vi "Build DashBoard Data.vi"(8 "finish":bool, 11 "Dashboard Enables":T3={"Analog Module 1"=[TRUE, TRUE, TRUE, TRUE, TRUE, TRUE, TRUE, TRUE], "Analog Module 2"=[FALSE, FALSE, FALSE, FALSE, FALSE, FALSE, FALSE, FALSE], "Digital Module 1"=TRUE, "Digital Module 2"=FALSE, "Solenoid Module"=TRUE}) -> ()   [LabVIEW 2011]
doc: "This VI builds data and sends it back to the dashboard PC program. By default it sends back the raw values for the first analog, digital, and solenoid module. Modify it to send back the data you want to view. Consider adding higher level data to the Dashboard Datatype.ctl and to this VI. Then update the Dashboard to display the data however you like.\n\nThis software is licensed. Open the labview\\readme\\WPI Robotics Library Open Source License.txt file for more information."
uses:
  DashboardEnable.ctl
  Dashboard Datatype.ctl
  <vilib>/Rock Robotics/WPI/DriverStation/WPI_DriverStationDigitalData.ctl
  Robot Global Data.vi
panel:
  out "Dashboard Data":T1
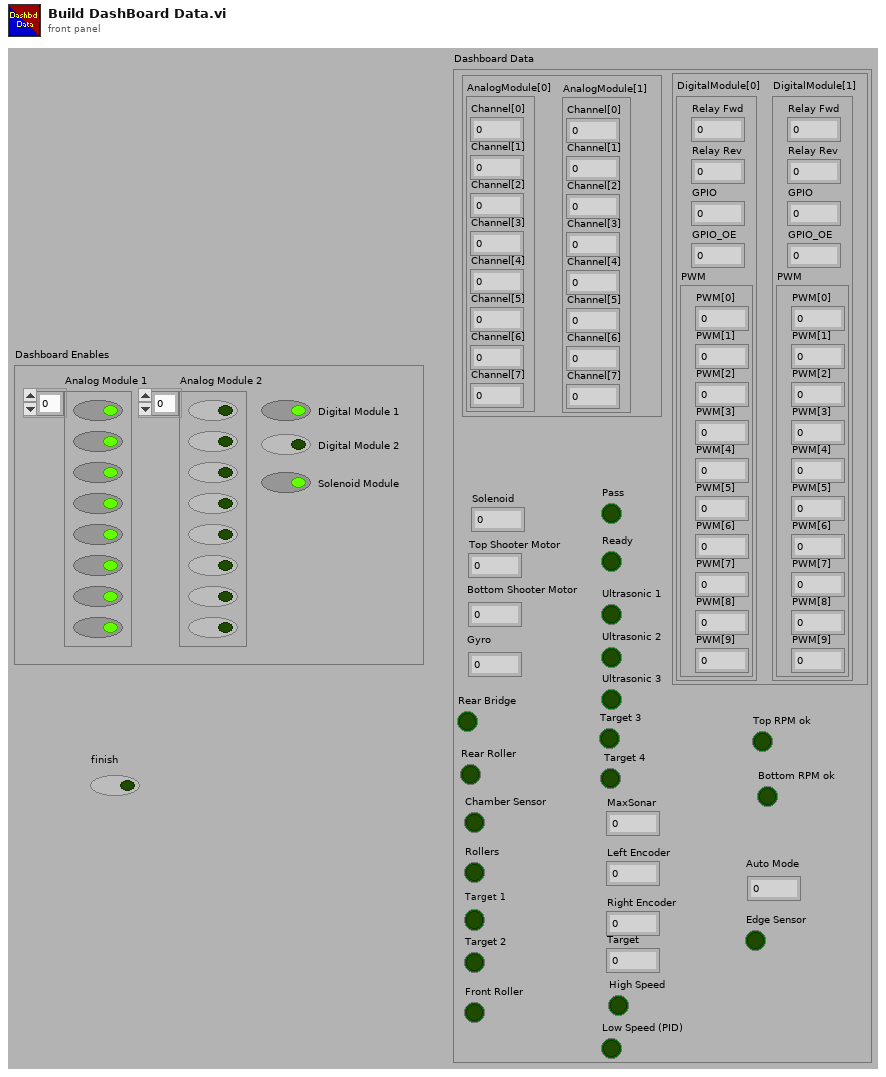
[diagram p1: front panel]
types:
  T1 = typedef "Dashboard Datatype.ctl" = cluster{cluster{"AnalogModule[0]":cluster{"Channel[0]":sgl, "Channel[1]":sgl, "Channel[2]":sgl, "Channel[3]":sgl, "Channel[4]":sgl, "Channel[5]":sgl, "Channel[6]":sgl, "Channel[7]":sgl}, "AnalogModule[1]":cluster{"Channel[0]":sgl, "Channel[1]":sgl, "Channel[2]":sgl, "Channel[3]":sgl, "Channel[4]":sgl, "Channel[5]":sgl, "Channel[6]":sgl, "Channel[7]":sgl}}, cluster{"DigitalModule[0]":T2, "DigitalModule[1]":T2}, "Solenoid":u8, "Top Shooter Motor":dbl, "Bottom Shooter Motor ":dbl, "Gyro":dbl, "Rear Roller":bool, "MaxSonar":dbl, "Left Encoder":dbl, "Right Encoder":dbl, "Chamber Sensor":bool, "Rear Bridge":bool, "Rollers":bool, "Target":dbl, "Target 1":bool, "Target 2":bool, " Target 4":bool, "Target 3":bool, "Pass":bool, "Ready":bool, "Ultrasonic 1":bool, "Ultrasonic 2":bool, "Ultrasonic 3":bool, "Front Roller":bool, "High Speed":bool, "Low Speed (PID)":bool, "Auto Mode":i16, "Top RPM ok":bool, "Bottom RPM ok":bool, "Edge Sensor":bool}
  T2 = typedef "WPI_DriverStationDigitalData.ctl" = cluster{"Relay Fwd":u8, "Relay Rev":u8, "GPIO":u16, "GPIO_OE":u16, "PWM":cluster{"PWM[0]":u8, "PWM[1]":u8, "PWM[2]":u8, "PWM[3]":u8, "PWM[4]":u8, "PWM[5]":u8, "PWM[6]":u8, "PWM[7]":u8, "PWM[8]":u8, "PWM[9]":u8}}
  T3 = typedef "DashboardEnable.ctl" = cluster{"Analog Module 1":bool[], "Analog Module 2":bool[], "Digital Module 1":bool, "Digital Module 2":bool, "Solenoid Module":bool}
  T4 = typedef "WPI_CounterDevRef.ctl" = cluster{"DevStatus":errorcluster, "CntIndex":T5}
  T5 = typedef "FPGA_CounterCtrSystemIndex.ctl" = enum8{"Ctr 0", "Ctr 1", "Ctr 2", "Ctr 3", "Ctr 4", "Ctr 5", "Ctr 6", "Ctr 7", "Invalid"}
  T6 = typedef "WPI_DigitalInputDevRef.ctl" = cluster{"DevStatus":errorcluster, "DIO Channel":T7, "Digital Module":T8}
  T7 = typedef "FPGA_DIOChannel.ctl" = enum8{"DIO 1", "DIO 2", "DIO 3", "DIO 4", "DIO 5", "DIO 6", "DIO 7", "DIO 8", "DIO 9", "DIO 10", "DIO 11", "DIO 12", "DIO 13", "DIO 14", "Invalid"}
  T8 = typedef "FPGA_TypedefDigitalModule.ctl" = enum16{"Digital Module 1", "Digital Module 2"}
  T9 = typedef "WPI_JoystickDevRef.ctl" = cluster{"Device":T10}
  T10 = typedef "WPI_JoystickDeviceEnum.ctl" = enum16{"USB 1", "USB 2", "USB 3", "USB 4", "Kinect 1", "Kinect 2"}
  T11 = typedef "WPI_JoystickButtonState.ctl" = cluster{"Button 1":bool, "Button 2":bool, "Button 3":bool, "Button 4":bool, "Button 5":bool, "Button 6":bool, "Button 7":bool, "Button 8":bool, "Button 9":bool, "Button 10":bool, "Button 11":bool, "Button 12":bool}
  T12 = typedef "WPI_GyroDevRef.ctl" = cluster{"DevStatus":errorcluster, "Analog Module":T13, "Analog Channel":T14, "Offset":dbl, "Gain (VoltsPerDegree/Second)":dbl}
  T13 = typedef "FPGA_TypedefAnalogModule.ctl" = enum16{"Analog Module 1", "Analog Module 2"}
  T14 = typedef "FPGA_AIChannel.ctl" = enum8{"AI 1", "AI 2", "AI 3", "AI 4", "AI 5", "AI 6", "AI 7", "AI 8", "Invalid"}
  T15 = cluster{"AnalogModule[0]":cluster{"Channel[0]":sgl, "Channel[1]":sgl, "Channel[2]":sgl, "Channel[3]":sgl, "Channel[4]":sgl, "Channel[5]":sgl, "Channel[6]":sgl, "Channel[7]":sgl}, "AnalogModule[1]":cluster{"Channel[0]":sgl, "Channel[1]":sgl, "Channel[2]":sgl, "Channel[3]":sgl, "Channel[4]":sgl, "Channel[5]":sgl, "Channel[6]":sgl, "Channel[7]":sgl}}
  T16 = cluster{"Channel[0]":sgl, "Channel[1]":sgl, "Channel[2]":sgl, "Channel[3]":sgl, "Channel[4]":sgl, "Channel[5]":sgl, "Channel[6]":sgl, "Channel[7]":sgl}[]
  T17 = cluster{"Channel[0]":sgl, "Channel[1]":sgl, "Channel[2]":sgl, "Channel[3]":sgl, "Channel[4]":sgl, "Channel[5]":sgl, "Channel[6]":sgl, "Channel[7]":sgl}
  T18 = cluster{"AnalogModule[0][0]":sgl, "AnalogModule[0][1]":sgl, "AnalogModule[0][2]":sgl, "AnalogModule[0][3]":sgl, "AnalogModule[0][4]":sgl, "AnalogModule[0][5]":sgl, "AnalogModule[0][6]":sgl, "AnalogModule[0][7]":sgl}
  T19 = cluster{"[0]":cluster{"Channel[0]":sgl, "Channel[1]":sgl, "Channel[2]":sgl, "Channel[3]":sgl, "Channel[4]":sgl, "Channel[5]":sgl, "Channel[6]":sgl, "Channel[7]":sgl}, "[1]":cluster{"Channel[0]":sgl, "Channel[1]":sgl, "Channel[2]":sgl, "Channel[3]":sgl, "Channel[4]":sgl, "Channel[5]":sgl, "Channel[6]":sgl, "Channel[7]":sgl}}
  T20 = cluster{"DigitalModule[0]":T2, "DigitalModule[1]":T2}
  T21 = typedef "FPGA_DIODevRef.ctl" = cluster{"DevStatus":errorcluster, "Module":T8}
  T22 = cluster{"[0]":u8, "[1]":u8, "[2]":u8, "[3]":u8, "[4]":u8, "[5]":u8, "[6]":u8, "[7]":u8, "[8]":u8, "[9]":u8}
  T23 = typedef "FPGA_SolenoidDevRef.ctl" = cluster{"DevStatus":errorcluster, "Module":T24}
  T24 = typedef "FPGA_TypedefSolenoidModule.ctl" = enum16{"Solenoid Module 1", "Solenoid Module 2"}
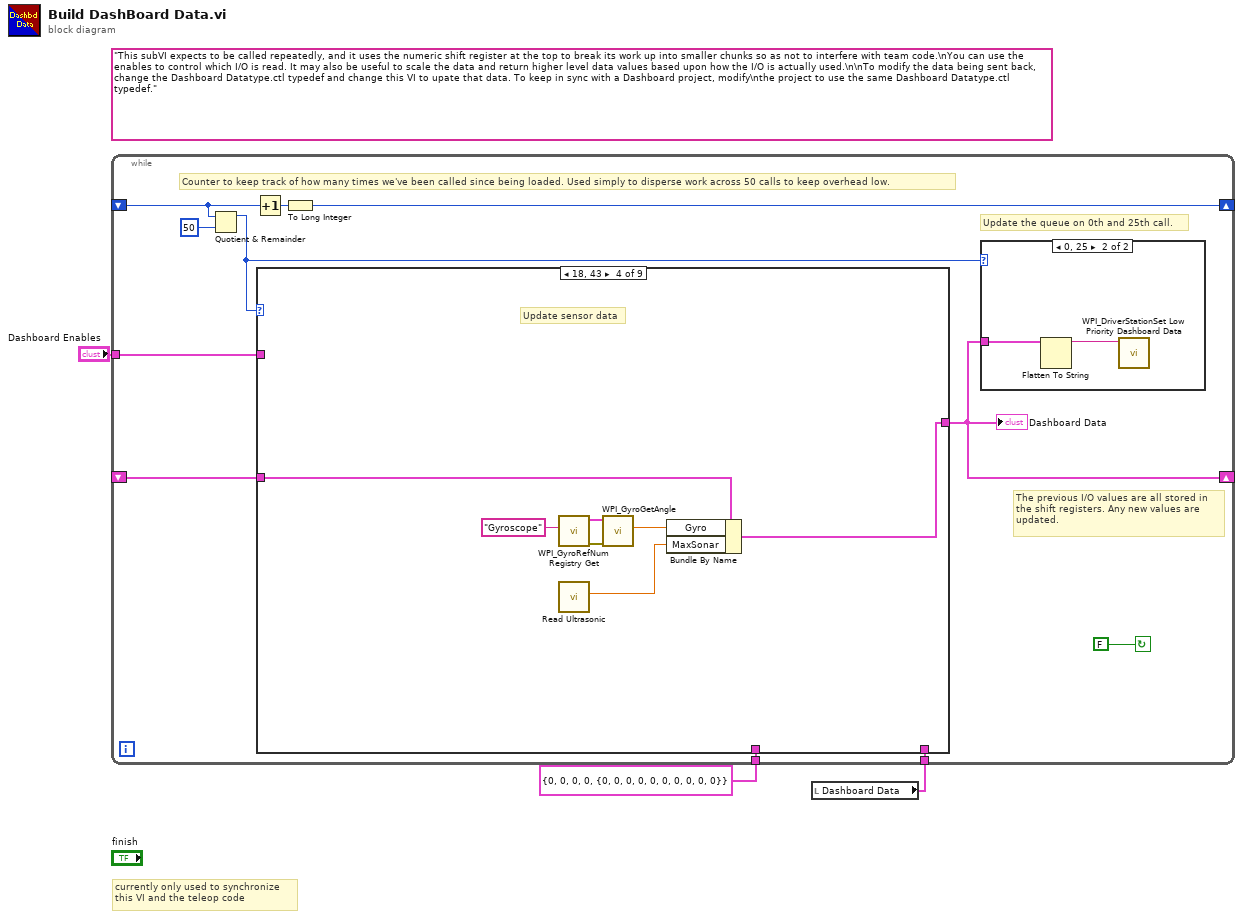
[diagram p0: block diagram]
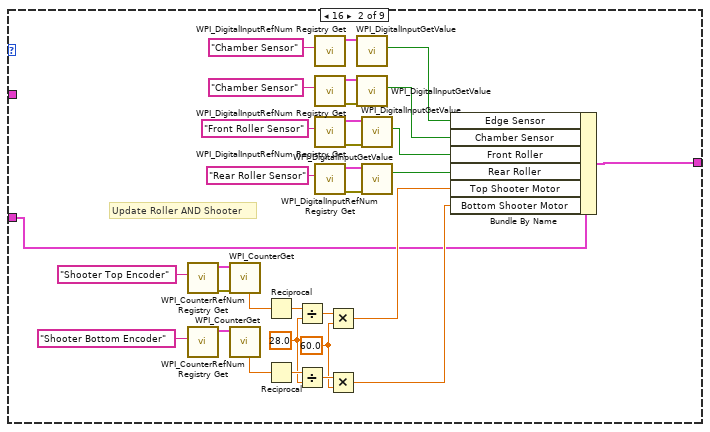
[diagram p4: hidden frame]
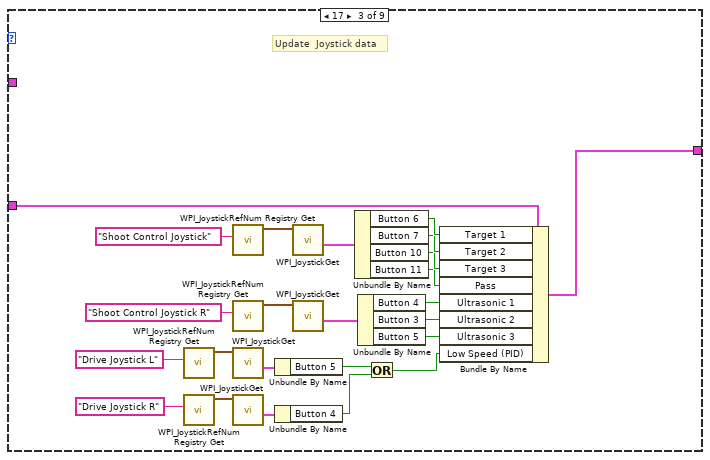
[diagram p5: hidden frame]
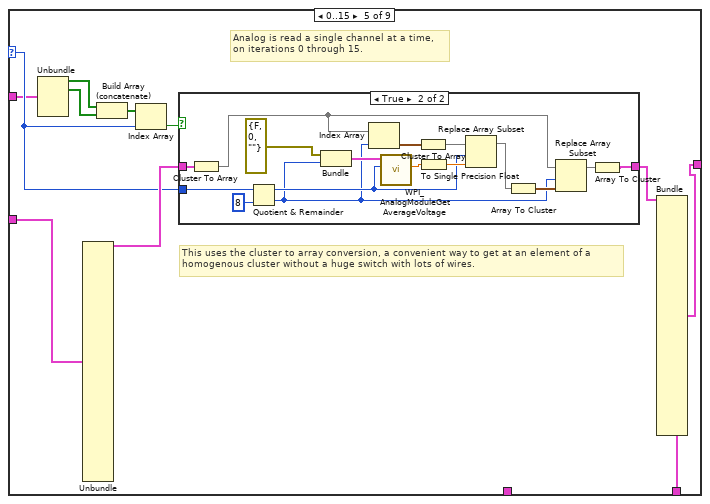
[diagram p6: hidden frame]
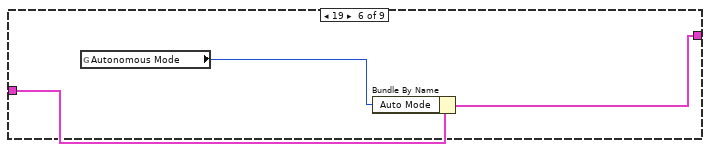
[diagram p8: hidden frame]
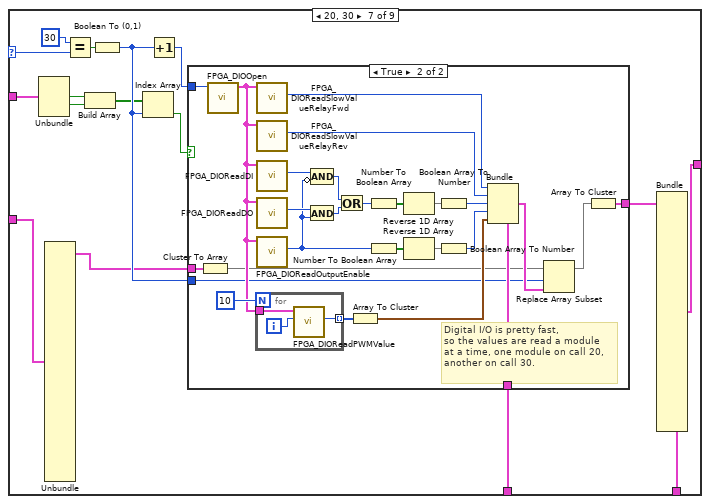
[diagram p9: hidden frame]
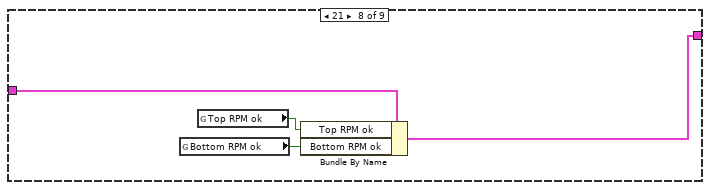
[diagram p11: hidden frame]
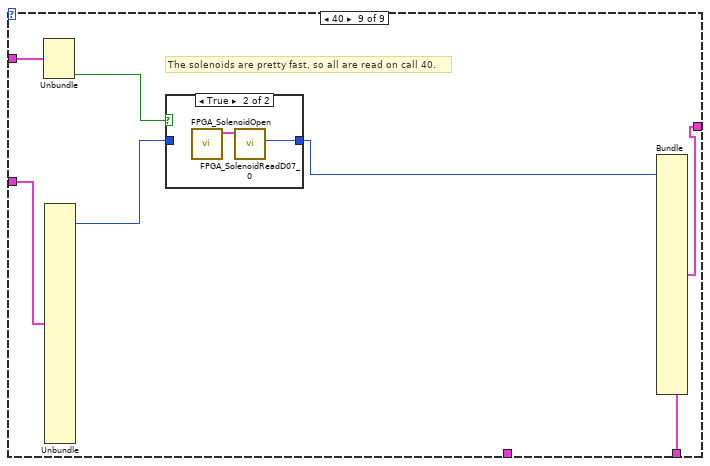
[diagram p12: hidden frame]
diagram:
  (unwired) "This subVI expects to be called repeatedly, and it uses the numeric shift register at the top to break its work up into smaller chunks so as not to interfere with team code.\nYou can use the enables to control which I/O is read. It may also be useful to scale the data and return higher level data values based upon how the I/O is actually used.\n\nTo modify the data being sent back, change the Dashboard Datatype.ctl typedef and change this VI to upate that data. To keep in sync with a Dashboard project, modify\nthe project to use the same Dashboard Datatype.ctl typedef."
  # "currently only used to synchronize\nthis VI and the teleop code"
  n1 = local read "Dashboard Data"() -> (w2:T1)
  n2 = while {
    shift-right: [w7] -> _
    shift-left: _ -> [w9]
    shift-right: [w4] -> _
    shift-left: _ -> [w12]
    tunnel: T2 {"Relay Fwd"=0, "Relay Rev"=0, "GPIO"=0, "GPIO_OE"=0, "PWM"={"PWM[0]"=0, "PWM[1]"=0, "PWM[2]"=0, "PWM[3]"=0, "PWM[4]"=0, "PWM[5]"=0, "PWM[6]"=0, "PWM[7]"=0, "PWM[8]"=0, "PWM[9]"=0}} ("DigitalModule[1]") -> [w11]
    tunnel: w2 -> [w6]
    tunnel: "Dashboard Enables" -> [w5]
    stop <- FALSE continue-if-true
    # "Counter to keep track of how many times we've been called since being loaded. Used simply to disperse work across 50 calls to keep overhead low."
    # "Update the queue on 0th and 25th call."
    # "The previous I/O values are all stored in\nthe shift registers. Any new values are\nupdated."
    n3 = Quotient & Remainder(x=w9, y=50) -> (x-y*floor(x/y)=w8:i32)  [unwired: 1 out]
    n4 = Increment(x=w9) -> (x+1=w14:i32)
    n5 = case shown="18, 43" w8 {
      selector: w8 -> [_ _ _ _ w86 _ w121 _ _]
      tunnel: [w17 w49 w72 w79 w82 w110 w112 w160 w165] -> w4
      tunnel: w12 -> [w17 w19 w73 w80 w81 w111 w114 w161 w167]
      tunnel: w11 -> [_ _ _ _ _ _ w127 _ _]
      tunnel: w6 -> [_ _ _ _ w88 _ w113 _ w164]
      tunnel: w5 -> [_ _ _ _ w85 _ w119 _ w168]
      frame Default {
        # "Don't update any I/O"
      }
      frame 16 {
        w27 = 60.0 ("y")
        w30 = 28.0 ("y")
        # "Update Roller AND Shooter"
        n6 = call <vilib>:"WPI_CounterRefNum Registry Get.vi"("refnum name"="Shooter Top Encoder") -> ("error out"=w37:errorcluster, "CounterDevRef"=w36:T4)  [unwired: 9 in]
        n7 = call <vilib>:"WPI_CounterRefNum Registry Get.vi"("refnum name"="Shooter Bottom Encoder") -> ("CounterDevRef"=w35:T4)  [unwired: 9 in, 1 out]
        n8 = call <vilib>:"WPI_CounterGet.vi"("error in (no error)"=w37, "CounterDevRef in"=w36) -> ("Period (sec)"=w34:dbl)  [unwired: 4 in, 5 out]
        n9 = call <vilib>:"WPI_CounterGet.vi"("CounterDevRef in"=w35) -> ("Period (sec)"=w33:dbl)  [unwired: 5 in, 5 out]
        n10 = Reciprocal(x=w34) -> (1/x=w31:dbl)
        n11 = Reciprocal(x=w33) -> (1/x=w32:dbl)
        n12 = Divide(x=w31, y=w30) -> (x/y=w29:dbl)
        n13 = Divide(x=w32, y=w30) -> (x/y=w28:dbl)
        n14 = call <vilib>:"WPI_DigitalInputRefNum Registry Get.vi"("refnum name"="Chamber Sensor") -> ("DigitalInputDevRef"=w21:T6)  [unwired: 9 in, 1 out]
        n15 = call <vilib>:"WPI_DigitalInputRefNum Registry Get.vi"("refnum name"="Chamber Sensor") -> ("error out"=w43:errorcluster, "DigitalInputDevRef"=w44:T6)  [unwired: 9 in]
        n16 = call <vilib>:"WPI_DigitalInputRefNum Registry Get.vi"("refnum name"="Front Roller Sensor") -> ("error out"=w48:errorcluster, "DigitalInputDevRef"=w47:T6)  [unwired: 9 in]
        n17 = call <vilib>:"WPI_DigitalInputRefNum Registry Get.vi"("refnum name"="Rear Roller Sensor") -> ("error out"=w40:errorcluster, "DigitalInputDevRef"=w41:T6)  [unwired: 9 in]
        n18 = Multiply(x=w29, y=w27) -> (x*y=w26:dbl)
        n19 = Multiply(x=w28, y=w27) -> (x*y=w25:dbl)
        n20 = call <vilib>:"WPI_DigitalInputGetValue.vi"("DigitalInputDevRef"=w21) -> ("Value"=w18:bool)  [unwired: 8 in, 2 out]
        n21 = call <vilib>:"WPI_DigitalInputGetValue.vi"("error in (no error)"=w43, "DigitalInputDevRef"=w44) -> ("Value"=w24:bool)  [unwired: 7 in, 2 out]
        n22 = call <vilib>:"WPI_DigitalInputGetValue.vi"("error in (no error)"=w48, "DigitalInputDevRef"=w47) -> ("Value"=w23:bool)  [unwired: 7 in, 2 out]
        n23 = call <vilib>:"WPI_DigitalInputGetValue.vi"("error in (no error)"=w40, "DigitalInputDevRef"=w41) -> ("Value"=w22:bool)  [unwired: 7 in, 2 out]
        n24 = Bundle By Name(cluster=w19, "Edge Sensor"=w18, "Chamber Sensor"=w24, "Front Roller"=w23, "Rear Roller"=w22, "Top Shooter Motor"=w26, "Bottom Shooter Motor"=w25) -> (w49:T1)
      }
      frame 17 {
        # "Update  Joystick data"
        n25 = call <vilib>:"WPI_JoystickRefNum Registry Get.vi"("refnum name"="Drive Joystick L") -> ("JoystickDevRef"=w58:T9)  [unwired: 9 in, 1 out]
        n26 = call <vilib>:"WPI_JoystickRefNum Registry Get.vi"("refnum name"="Drive Joystick R") -> ("JoystickDevRef"=w55:T9)  [unwired: 9 in, 1 out]
        n27 = call <vilib>:"WPI_JoystickRefNum Registry Get.vi"("refnum name"="Shoot Control Joystick") -> ("JoystickDevRef"=w69:T9)  [unwired: 9 in, 1 out]
        n28 = call <vilib>:"WPI_JoystickRefNum Registry Get.vi"("refnum name"="Shoot Control Joystick R") -> ("JoystickDevRef"=w62:T9)  [unwired: 9 in, 1 out]
        n29 = call <vilib>:"WPI_JoystickGet.vi"("JoystickDevRef"=w58) -> ("Buttons"=w53:T11)  [unwired: 4 in, 2 out]
        n30 = call <vilib>:"WPI_JoystickGet.vi"("JoystickDevRef"=w55) -> ("Buttons"=w54:T11)  [unwired: 4 in, 2 out]
        n31 = Unbundle By Name(w53) -> ("Button 5"=w51:bool)
        n32 = Unbundle By Name(w54) -> ("Button 4"=w52:bool)
        n33 = call <vilib>:"WPI_JoystickGet.vi"("JoystickDevRef"=w69) -> ("Buttons"=w71:T11)  [unwired: 4 in, 2 out]
        n34 = call <vilib>:"WPI_JoystickGet.vi"("JoystickDevRef"=w62) -> ("Buttons"=w64:T11)  [unwired: 4 in, 2 out]
        n35 = Unbundle By Name(w71) -> ("Button 6"=w68:bool, "Button 7"=w67:bool, "Button 10"=w66:bool, "Button 11"=w65:bool)
        n36 = Unbundle By Name(w64) -> ("Button 4"=w61:bool, "Button 3"=w60:bool, "Button 5"=w59:bool)
        n37 = Or(x=w51, y=w52) -> (x .or. y?=w50:bool)
        n38 = Bundle By Name(cluster=w73, "Target 1"=w68, "Target 2"=w67, "Target 3"=w66, "Pass"=w65, "Ultrasonic 1"=w61, "Ultrasonic 2"=w60, "Ultrasonic 3"=w59, "Low Speed (PID)"=w50) -> (w72:T1)
      }
      frame 18, 43 {
        # "Update sensor data"
        n39 = call <vilib>:"WPI_GyroRefNum Registry Get.vi"("refnum name"="Gyroscope") -> ("error out"=w76:errorcluster, "GyroDevRef"=w77:T12)  [unwired: 9 in]
        n40 = call "Read Ultrasonic.vi"() -> ("distance"=w74:dbl)  [unwired: 11 in]
        n41 = call <vilib>:"WPI_GyroGetAngle.vi"("error in (no error)"=w76, "GyroDevRef"=w77) -> ("Angle"=w75:dbl)  [unwired: 6 in, 3 out]
        n42 = Bundle By Name(cluster=w80, "Gyro"=w75, "MaxSonar"=w74) -> (w79:T1)
      }
      frame 0..15 {
        # "This uses the cluster to array conversion, a convenient way to get at an element of a\nhomogenous cluster without a huge switch with lots of wires."
        # "Analog is read a single channel at a time,\non iterations 0 through 15."
        n43 = Unbundle(w85) -> ("Analog Module 1"=w84:bool[], "Analog Module 2"=w83:bool[])  [unwired: 3 out]
        n44 = Unbundle(w81) -> (w87:T15)  [unwired: 29 out]
        n45 = Build Array (concatenate)(w84, w83) -> (w90:bool[])
        n46 = Index Array(array=w90, index=w86) -> (element=w91:bool)
        n47 = case shown="True" w91 {
          tunnel: w86 -> [_ w99]
          tunnel: [w92 w96] -> w89
          tunnel: w87 -> [w92 w95]
          frame False {
          }
          frame True {
            n48 = Cluster To Array(cluster=w95) -> (array=w94:T16)
            n49 = Quotient & Remainder(x=w99, y=8) -> (x-y*floor(x/y)=w98:i32, floor(x/y)=w93:i32)
            n50 = Bundle("DevStatus"=errorcluster {"status"=FALSE, "code"=0, "source"=""}, w93) -> (w107:cluster{"DevStatus":errorcluster, i32})  [unwired: 1 out]
            n51 = Index Array(array=w94, index=w93) -> (element=w101:T17)
            n52 = call <vilib>:"WPI_AnalogModuleGetAverageVoltage.vi"("Channel"=w98, "AnalogModuleDevStatus"=w107) -> ("Average Voltage"=w104:dbl)  [unwired: 1 in, 8 out]
            n53 = Cluster To Array(cluster=w101) -> (array=w100:sgl[])
            n54 = To Single Precision Float(number=w104) -> (single precision float=w103:sgl)
            n55 = Replace Array Subset(array=w100, new element=w103, index=w98) -> (w102:sgl[])
            n56 = Array To Cluster(array=w102) -> (cluster=w106:T18)
            n57 = Replace Array Subset(array=w94, new element=w106, index=w93) -> (w97:T16)
            n58 = Array To Cluster(array=w97) -> (cluster=w96:T19)
          }
        }
        n59 = Bundle(cluster=w88, w89) -> (w82:T1)  [unwired: 29 out]
      }
      frame 19 {
        n60 = global read "Robot Global Data.vi" "Autonomous Mode"() -> (w109:i16)
        n61 = Bundle By Name(cluster=w111, "Auto Mode"=w109) -> (w110:T1)
      }
      frame 20, 30 {
        n62 = Unbundle(w119) -> ("Digital Module 1"=w118:bool, "Digital Module 2"=w117:bool)  [unwired: 3 out]
        n63 = Unbundle(w114) -> (w116:T20)  [unwired: 29 out]
        n64 = Equal?(x=30, y=w121) -> (x = y?=w125:bool)
        n65 = Build Array(w118, w117) -> (w120:bool[])
        n66 = Boolean To (0,1)(Boolean=w125) -> (0, 1=w123:i16)
        n67 = Index Array(array=w120, index=w123) -> (element=w122:bool)
        n68 = Increment(x=w123) -> (x+1=w124:i16)
        n69 = case shown="True" w122 {
          tunnel: w127 -> [_ w136]
          tunnel: [w128 w129] -> w115
          tunnel: w124 -> [_ w134]
          tunnel: w123 -> [_ w133]
          tunnel: w116 -> [w128 w132]
          frame False {
          }
          frame True {
            # "Digital I/O is pretty fast,\nso the values are read a module\nat a time, one module on call 20,\nanother on call 30."
            n70 = Cluster To Array(cluster=w132) -> (array=w131:T2[])
            n71 = call <vilib>:"FPGA_DIOOpen.vi"("Module (Module 1)"=w134) -> ("DIODeviceRef"=w152:T21)  [unwired: 1 in, 9 out]
            n72 = for {
              N: 10 -> [_]
              tunnel: w152 -> [w157]
              tunnel: [w155] -> w153 mode=indexing
              i -> [w156]
              n73 = call <vilib>:"FPGA_DIOReadPWMValue.vi"("PWMChannel"=w156, "DIODeviceRef In"=w157) -> ("PWMValue"=w155:u8)  [unwired: 1 in, 8 out]
            }
            n74 = call <vilib>:"FPGA_DIOReadSlowValueRelayFwd.vi"("DIODeviceRef In"=w152) -> ("Relay Forward"=w145:u8)  [unwired: 1 in, 9 out]
            n75 = call <vilib>:"FPGA_DIOReadSlowValueRelayRev.vi"("DIODeviceRef In"=w152) -> ("Relay Reverse"=w146:u8)  [unwired: 1 in, 9 out]
            n76 = call <vilib>:"FPGA_DIOReadDI.vi"("DIODeviceRef In"=w152) -> ("DI"=w150:u16)  [unwired: 1 in, 9 out]
            n77 = call <vilib>:"FPGA_DIOReadDO.vi"("DIODeviceRef In"=w152) -> ("DO"=w149:u16)  [unwired: 1 in, 9 out]
            n78 = call <vilib>:"FPGA_DIOReadOutputEnable.vi"("DIODeviceRef In"=w152) -> ("OutputEnable"=w140:u16)  [unwired: 1 in, 9 out]
            n79 = And(x=w149, y=w140) -> (x .and. y?=w148:u16)
            n80 = Compound Arithmetic op=AND(w150, invert w140) -> (w147:u16)
            n81 = Or(x=w147, y=w148) -> (x .or. y?=w138:u16)
            n82 = Array To Cluster(array=w153) -> (cluster=w151:T22)
            n83 = Number To Boolean Array(number=w138) -> (Boolean array=w143:bool[])
            n84 = Number To Boolean Array(number=w140) -> (Boolean array=w142:bool[])
            n85 = Reverse 1D Array(array=w143) -> (reversed array=w144:bool[])
            n86 = Reverse 1D Array(array=w142) -> (reversed array=w141:bool[])
            n87 = Boolean Array To Number(Boolean array=w144) -> (number=w137:u32)
            n88 = Boolean Array To Number(Boolean array=w141) -> (number=w139:u32)
            n89 = Bundle(cluster=w136, "Relay Fwd"=w145, "Relay Rev"=w146, "GPIO"=w137, "GPIO_OE"=w139, "PWM"=w151) -> (w135:T2)
            n90 = Replace Array Subset(array=w131, new element=w135, index=w133) -> (w130:T2[])
            n91 = Array To Cluster(array=w130) -> (cluster=w129:cluster{"[0]":T2, "[1]":T2})
          }
        }
        n92 = Bundle(cluster=w113, w115) -> (w112:T1)  [unwired: 29 out]
      }
      frame 21 {
        n93 = global read "Robot Global Data.vi" "Bottom RPM ok"() -> (w158:bool)
        n94 = global read "Robot Global Data.vi" "Top RPM ok"() -> (w159:bool)
        n95 = Bundle By Name(cluster=w161, "Top RPM ok"=w159, "Bottom RPM ok"=w158) -> (w160:T1)
      }
      frame 40 {
        # "The solenoids are pretty fast, so all are read on call 40."
        n96 = Unbundle(w168) -> ("Solenoid Module"=w162:bool)  [unwired: 4 out]
        n97 = Unbundle(w167) -> ("Solenoid"=w166:u8)  [unwired: 29 out]
        n98 = case shown="True" w162 {
          tunnel: [w169 w170] -> w163
          tunnel: w166 -> [w169 _]
          frame False {
          }
          frame True {
            n99 = call <vilib>:"FPGA_SolenoidOpen.vi"() -> ("SolenoidDevRef"=w171:T23)  [unwired: 2 in, 9 out]
            n100 = call <vilib>:"FPGA_SolenoidReadD07_0.vi"("SolenoidDevRef"=w171) -> ("DO7:0"=w170:u8)  [unwired: 1 in, 9 out]
          }
        }
        n101 = Bundle(cluster=w164, "Solenoid"=w163) -> (w165:T1)  [unwired: 29 out]
      }
    }
    "Dashboard Data" <- w4
    n102 = To Long Integer(number=w14) -> (32bit integer=w7:i32)
    n103 = case shown="0, 25" w8 {
      tunnel: w4 -> [_ w16]
      frame Default {
      }
      frame 0, 25 {
        n104 = Flatten To String(anything=w16) -> (data string=w15:string)  [unwired: 1 in, 4 out]
        n105 = call <vilib>:"WPI_DriverStationSet Low Priority Dashboard Data.vi"("User Data"=w15) -> ()  [unwired: 1 in, 10 out]
      }
    }
  }
